vi "TPNT_WriteHTMLLog.vi"(6 "UTC":bool, 8 "error in (no error)":errorcluster, 9 "time format":string="%Y-%m-%dT%H:%M:%S", 10 "message":string, 11 "File":path) -> (0 "error out":errorcluster)   [LabVIEW 2016]
uses:
  <vilib>/Utility/NIReport.llb/Append Report Text (str wrap).vi
  <vilib>/Utility/NIReport.llb/NI_report.lvclass
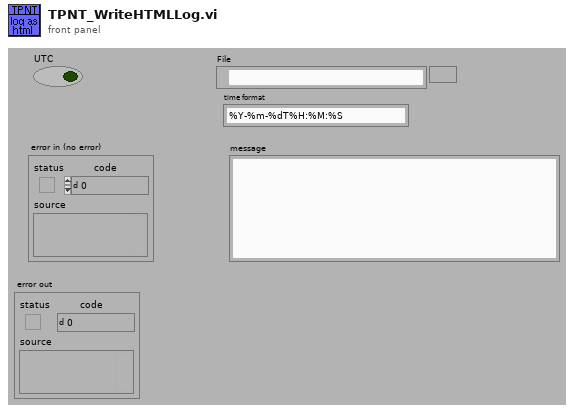
[diagram p1: front panel]
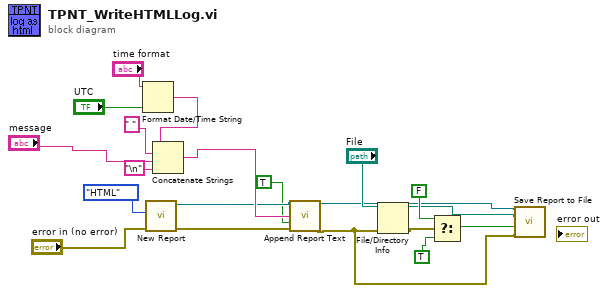
[diagram p0: block diagram]
diagram:
  n1 = Format Date/Time String(time format string (%c)="time format", UTC format="UTC") -> (date/time string=w18:string)  [unwired: 1 out]
  n2 = call <vilib>:"New Report.vi"("report type"=enum16{"Standard Report", "HTML"}."HTML", "error in (no error)"="error in (no error)") -> ("report out"=w12:refnum<class "NI_report.lvclass">, "error out"=w10:errorcluster)  [unwired: 4 in, 8 out]
  n3 = Concatenate Strings(w18, " ", "message", "\n") -> (w20:string)
  n4 = call-poly <vilib>:"Append Report Text.vi"("report in"=w12, "text"=w20, "append on new line? (F)"=TRUE, "error in (no error)"=w10) -> ("report out"=w4:refnum<class "NI_report.lvclass">, "error out"=w5:errorcluster)  [unwired: 2 in, 8 out]
  n5 = File/Directory Info(path="File", error in=w5) -> (path out=w3:path, error out=w9:errorcluster)  [unwired: 5 out]
  n6 = Select(t=FALSE, s=w9, f=TRUE) -> (s? t:f=w2:bool)
  n7 = call-dynamic "Save Report to File.vi"("report in"=w4, "report file path"=w3, "prompt to replace? (F)"=w2, "error in (no error)"=w5) -> ()  [unwired: 1 in, 11 out]
